vi "Read Text.vi"(9 "IOName in":refnum<class "IOName.lvclass">) -> (3 "IOName out":refnum<class "IOName.lvclass">, 4 "Text":refnum<class "Text.lvclass">)   [LabVIEW 2014, in "IOName.lvclass"]
uses:
  IOName.lvclass
  Text/Text.lvclass
  IOName.lvclass/IOName.ctl
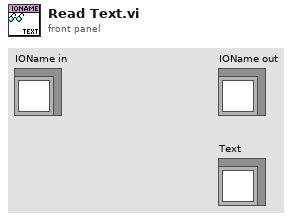
[diagram p1: front panel]
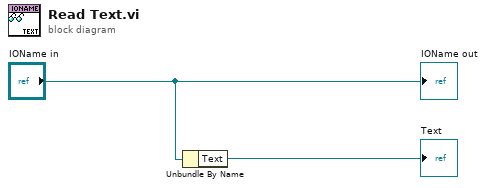
[diagram p0: block diagram]
diagram:
  n1 = Unbundle By Name("IOName in") -> ("Text"=→"Text":refnum<class "Text.lvclass">)
  "IOName out" <- "IOName in"
